vi "GetBmuNo.vi"(1 "类型":u32(ring)=4 items=["PCI5121"=1, "PCI9810"=2, "USBCAN1"=3, "USBCAN2"=4, "PCI9820"=5, "CAN232"=6, "PCI5110"=7, "CANLite(mini)"=8, "ISA9620"=9, "ISA5420"=10, "PC104CAN"=11, "CANET"=17, "DNP9810"=13, "USBCAN-E-U"=20, "USBCAN-2E-U"=21], 2 "设备索引":u32(ring) items=["0", "1", "2", "3", "4", "5", "6", "7", "8", "9", "10", "11", "12", "13", "14", "15", ""], 3 "CAN路数":u32(ring) items=["0", "1"], 11 "time out":u32) -> (4 "recv ok?":bool, 6 "BMU NO":u32)   [LabVIEW 2013]
uses:
  BMS_BootLoader/trunk/BMS_Bootloader/AutoBurn/Settings/ControlCAN.dll
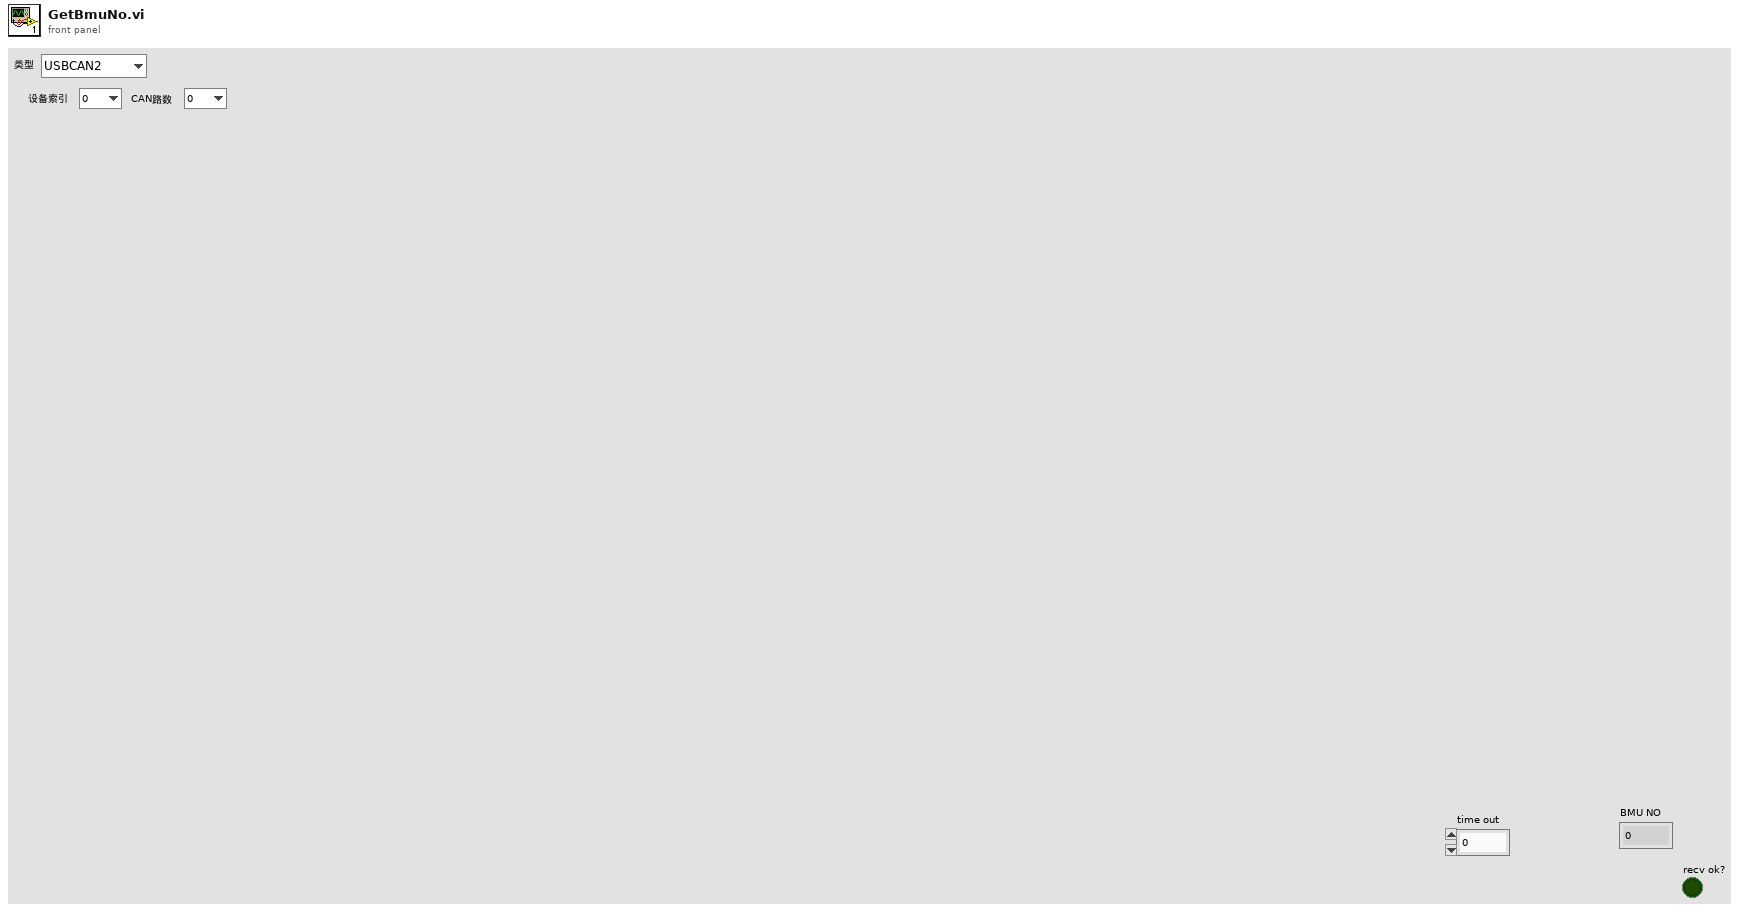
[diagram p1: front panel]
types:
  T1 = cluster{"ID":u32, "TimeStamp":u32, "TimeFlag":u8, "SendType":u8, "RemoteFlag":u8, "ExternFlag":u8, "DataLen":u8, u8, u8, u8, u8, u8, u8, u8, u8, u8, u8, u8}
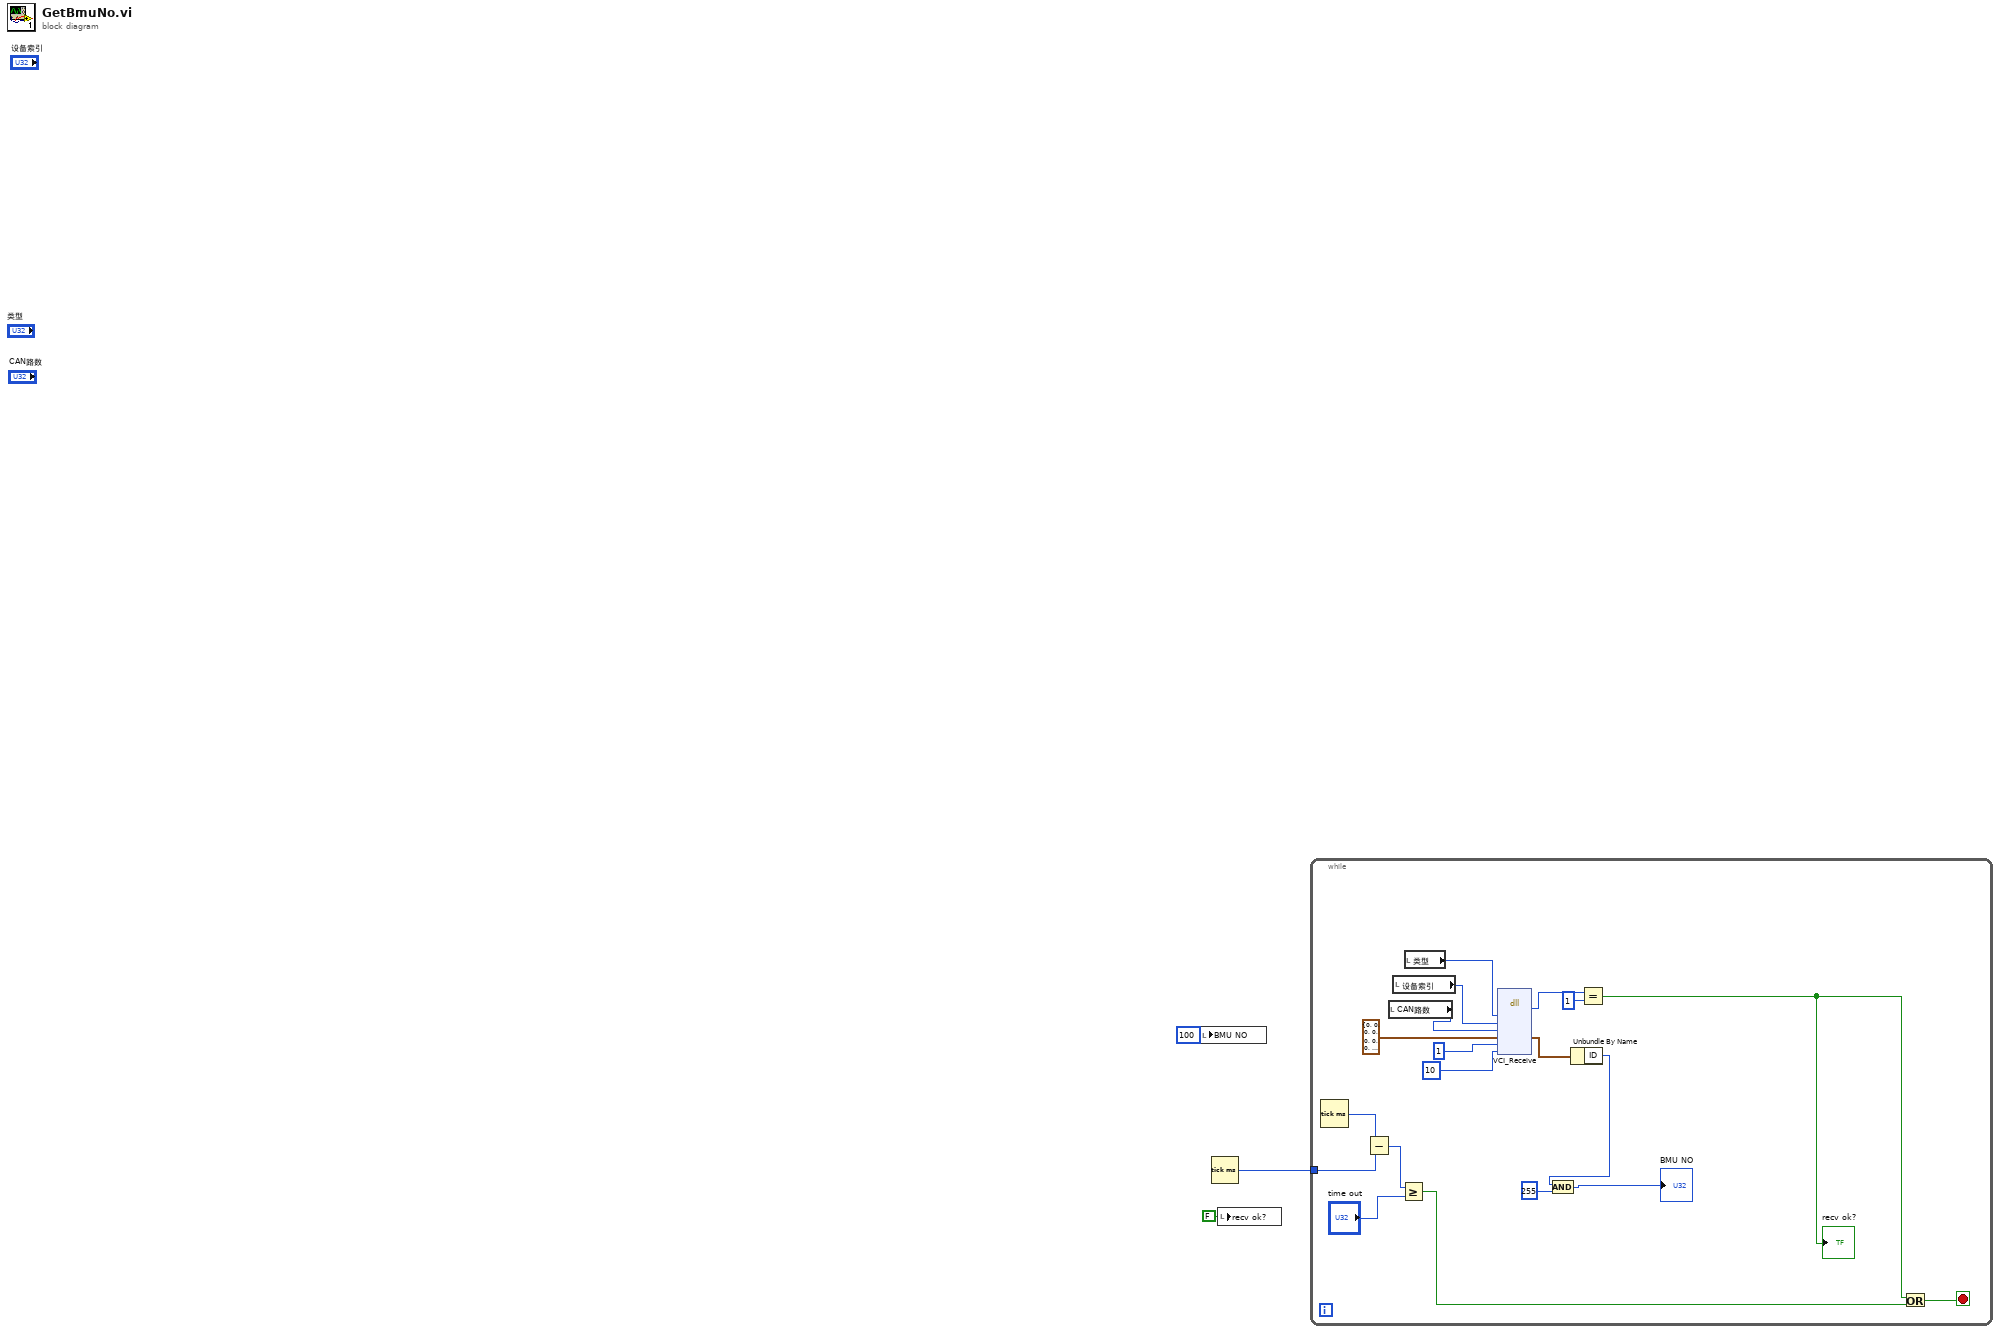
[diagram p0: block diagram]
diagram:
  n1 = local write "BMU NO"(u64 100 ("Value")) -> ()
  n2 = Tick Count (ms)() -> (millisecond timer value=w3:u32)
  n3 = local write "recv ok?"(FALSE ("x = y?")) -> ()
  n4 = while {
    tunnel: w3 -> [w15]
    stop <- w11 stop-if-true
    n5 = Tick Count (ms)() -> (millisecond timer value=w16:u32)
    n6 = Subtract(x=w16, y=w15) -> (x-y=w14:u32)
    n7 = local read "CAN路数"() -> (w20:u32)
    n8 = local read "设备索引"() -> (w17:u32)
    n9 = Greater Or Equal?(x=w14, y="time out") -> (x >= y?=w12:bool)
    n10 = local read "类型"() -> (w18:u32)
    n11 = dll-call lib="F:/Bluewave New Energy/SVN_Work/BMS_BootLoader/trunk/BMS_Bootloader/AutoBurn/Settings/ControlCAN.dll" fn="VCI_Receive"("DeviceType"=w18, "DeviceInd"=w17, "CANInd"=w20, "pReceive"=T1 {"ID"=0, "TimeStamp"=0, "TimeFlag"=0, "SendType"=0, "RemoteFlag"=0, "ExternFlag"=0, "DataLen"=0, 0, 0, 0, 0, 0, 0, 0, 0, 0, 0, 0}, "Len"=u32 1, "WaitTime"=10) -> ("返回类型"=w10:u32, "pReceive"=w6:T1)  [unwired: 8 in, 2 out]
    n12 = Unbundle By Name(w6) -> ("ID"=w5:u32)
    n13 = And(x=w5, y=u32 255) -> (x .and. y?=→"BMU NO":u32)
    n14 = Equal?(x=w10, y=u32 1) -> (x = y?=w8:bool)
    "recv ok?" <- w8
    n15 = Or(x=w8, y=w12) -> (x .or. y?=w11:bool)
  }
